vi "Фронт Д.vi"(2 "C":bool, 3 "S":bool, 4 "D":bool, 5 "R":bool) -> (0 "NOT Q":bool, 1 "Q":bool)   [LabVIEW 2017]
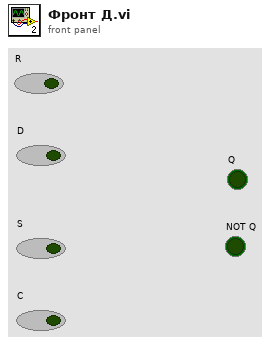
[diagram p1: front panel]
types:
  T1 = cluster{"R":bool, "  Q":bool, "S":bool, "C":bool}
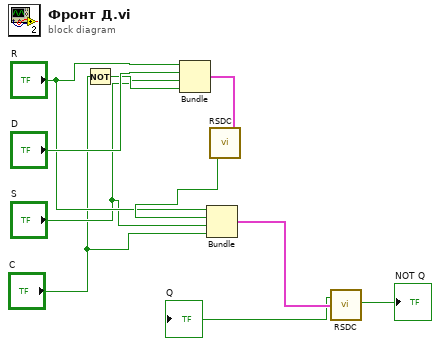
[diagram p0: block diagram]
diagram:
  n1 = Not(x="C") -> (.not. x?=w9:bool)
  n2 = Bundle("R"="R", "D"="D", "S"="S", w9) -> (w8:cluster{"R":bool, "D":bool, "S":bool, bool})  [unwired: 1 in]
  n3 = call "RSDC.vi"("Cluster"=w8) -> ("Q"=w7:bool)  [unwired: 1 out]
  n4 = Bundle("R"="R", "Q"=w7, "S"="S", "C"="C") -> (w3:T1)  [unwired: 1 in]
  n5 = call "RSDC.vi"("Cluster"=w3) -> ("-Q"=→"NOT Q":bool, "Q"=→"Q":bool)
